vi "Sistema de ventilación-Ramirez.vi"() -> ()   [LabVIEW 2023]
uses:
  <vilib>/MakerHub/LINX/Public/Peripherals/Analog/Analog Read 1 Chan.vi
  <vilib>/MakerHub/LINX/Public/Peripherals/Digital/Digital Write 1 Chan.vi
  <vilib>/MakerHub/LINX/Public/Peripherals/Analog/Analog Read N Chans.vi
  <vilib>/MakerHub/LINX/Public/Peripherals/Digital/Digital Write N Chans.vi
  <vilib>/MakerHub/LINX/Private/Local IO/LinxAnalogRead.vi
  <vilib>/MakerHub/LINX/Public/Utilities/Check Channel.vi
  <vilib>/MakerHub/LINX/Private/Local IO/LinxDigitalWrite.vi
  <vilib>/MakerHub/LINX/Public/Utilities/Open Serial.vi
  <vilib>/MakerHub/LINX/Public/Sensors/Motion/Servo/Servo Open One Channel.vi
  <vilib>/MakerHub/LINX/Public/Peripherals/Analog/Analog Write 1 Chan.vi
  <vilib>/MakerHub/LINX/Private/Utilties/Generate Error.vi
  <vilib>/MakerHub/LINX/Public/Sensors/Motion/Servo/Servo Set Pulse Width One Channel.vi
  <vilib>/MakerHub/LINX/Public/Sensors/Motion/Servo/Servo Close One Channel.vi
  <vilib>/MakerHub/LINX/LMH-LINX.lvlib
  <vilib>/MakerHub/LINX/Public/Sensors/Motion/Servo/Servo.lvlib
panel:
  out "?":bool
  out "?":bool
  out "?":bool
  out "?":bool
  in  "?":bool
  out "Serevo Aire Angulo":string
  out "Serevo Temp Angulo":string
  in  "Serial Port":refnum<visa-resource-name>
  out "?":bool
  out "?":bool
  out "?":bool
  out "?":bool
  out "?":bool
  out "?":bool
  out "?":bool
  out "?":bool
  out "?":bool
  out "?":bool
  out "?":bool
  out "?":bool
  out "?":bool
  out "?":bool
  out "?":bool
  out "?":bool
  out "?":bool
  out "?":bool
  in  "?":bool
  out "Filtro de Calor":bool
  out "Filtro de Aire":bool
  out "Ppm del aire":dbl(knob) scale=0.0..1800.0
  out "Temperatura":dbl(slide) scale=0.0..60.0
  out "t [sec]":dbl
  out "Iteration No":i32
  in  "?":bool
  out "VI is running?":bool caption="ON/OFF"
  # "SISTEMA DE VENTILACIÓN DE DOBLE FLUJO"
  # "Temperatura"
  # "Entrada"
  # "Calidad del aire"
  # "Salida"
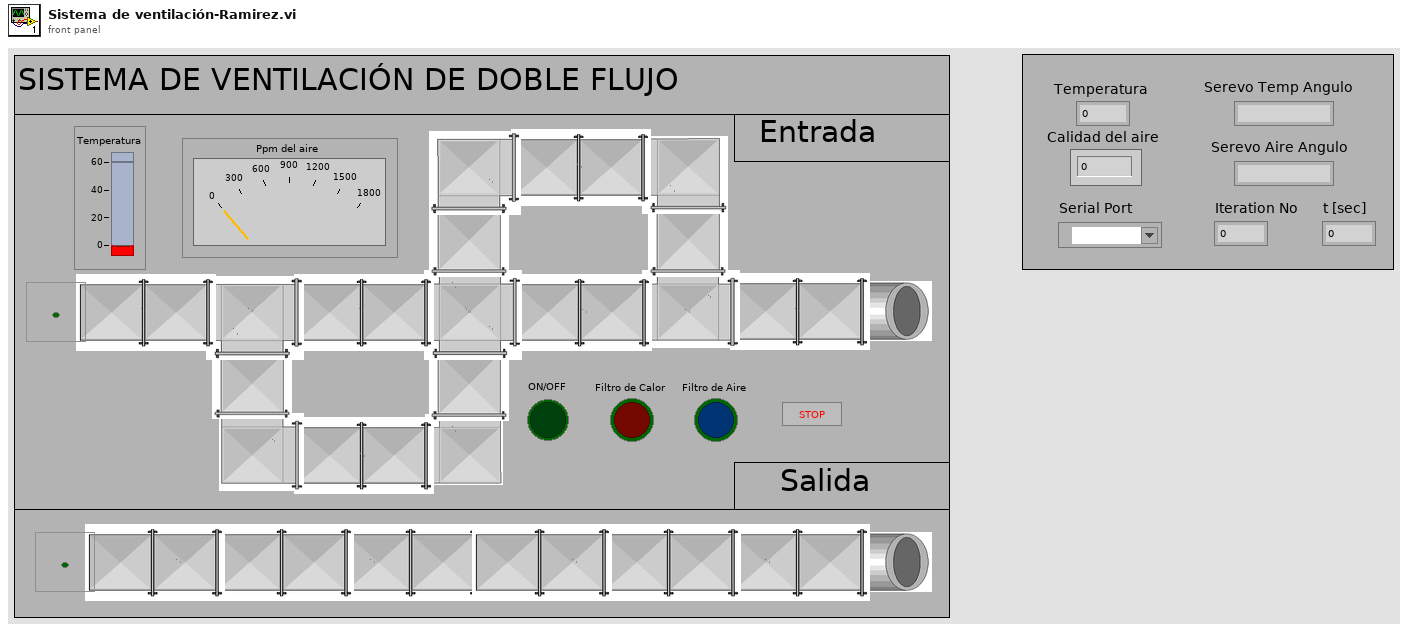
[diagram p1: front panel]
types:
  T1 = typedef "LMH-LINX.lvlib/LINX Ref.ctl" = cluster{"IO":T2, "Interface":T3, "LINX Device Config":T4}
  T2 = typedef "LMH-LINX.lvlib/Platform.ctl" = enum16{"Remote", "Local"}
  T3 = typedef "LMH-LINX.lvlib/Interface.ctl" = enum16{"Serial", "TCP"}
  T4 = typedef "LMH-LINX.lvlib/Device.lvlib/LINX Device Config.ctl" = cluster{"Interface":T3, "COM Port":refnum<visa-resource-name>, "TCP Configuration":T5, "Device Family":u8, "Device ID":u8, "Device Name":string, "TCP Ref":refnum<k5>, "Channels":T6}
  T5 = typedef "LMH-LINX.lvlib/Device.lvlib/TCP Config.ctl" = cluster{"IP Address":string, "Port":u16}
  T6 = typedef "LMH-LINX.lvlib/Channels.ctl" = cluster{"DI":u8[], "DO":u8[], "AI":u8[], "AO":u8[], "PWM":u8[], "QE":u8[], "UART":u8[], "I2C 2":u8[], "SPI":u8[], "CAN":u8[], "Servo":u8[], "AI Ref (V)":dbl, "AI Resolution (Bits)":u8, "AO Ref (V)":dbl, "AO Resolution (Bits)":u8}
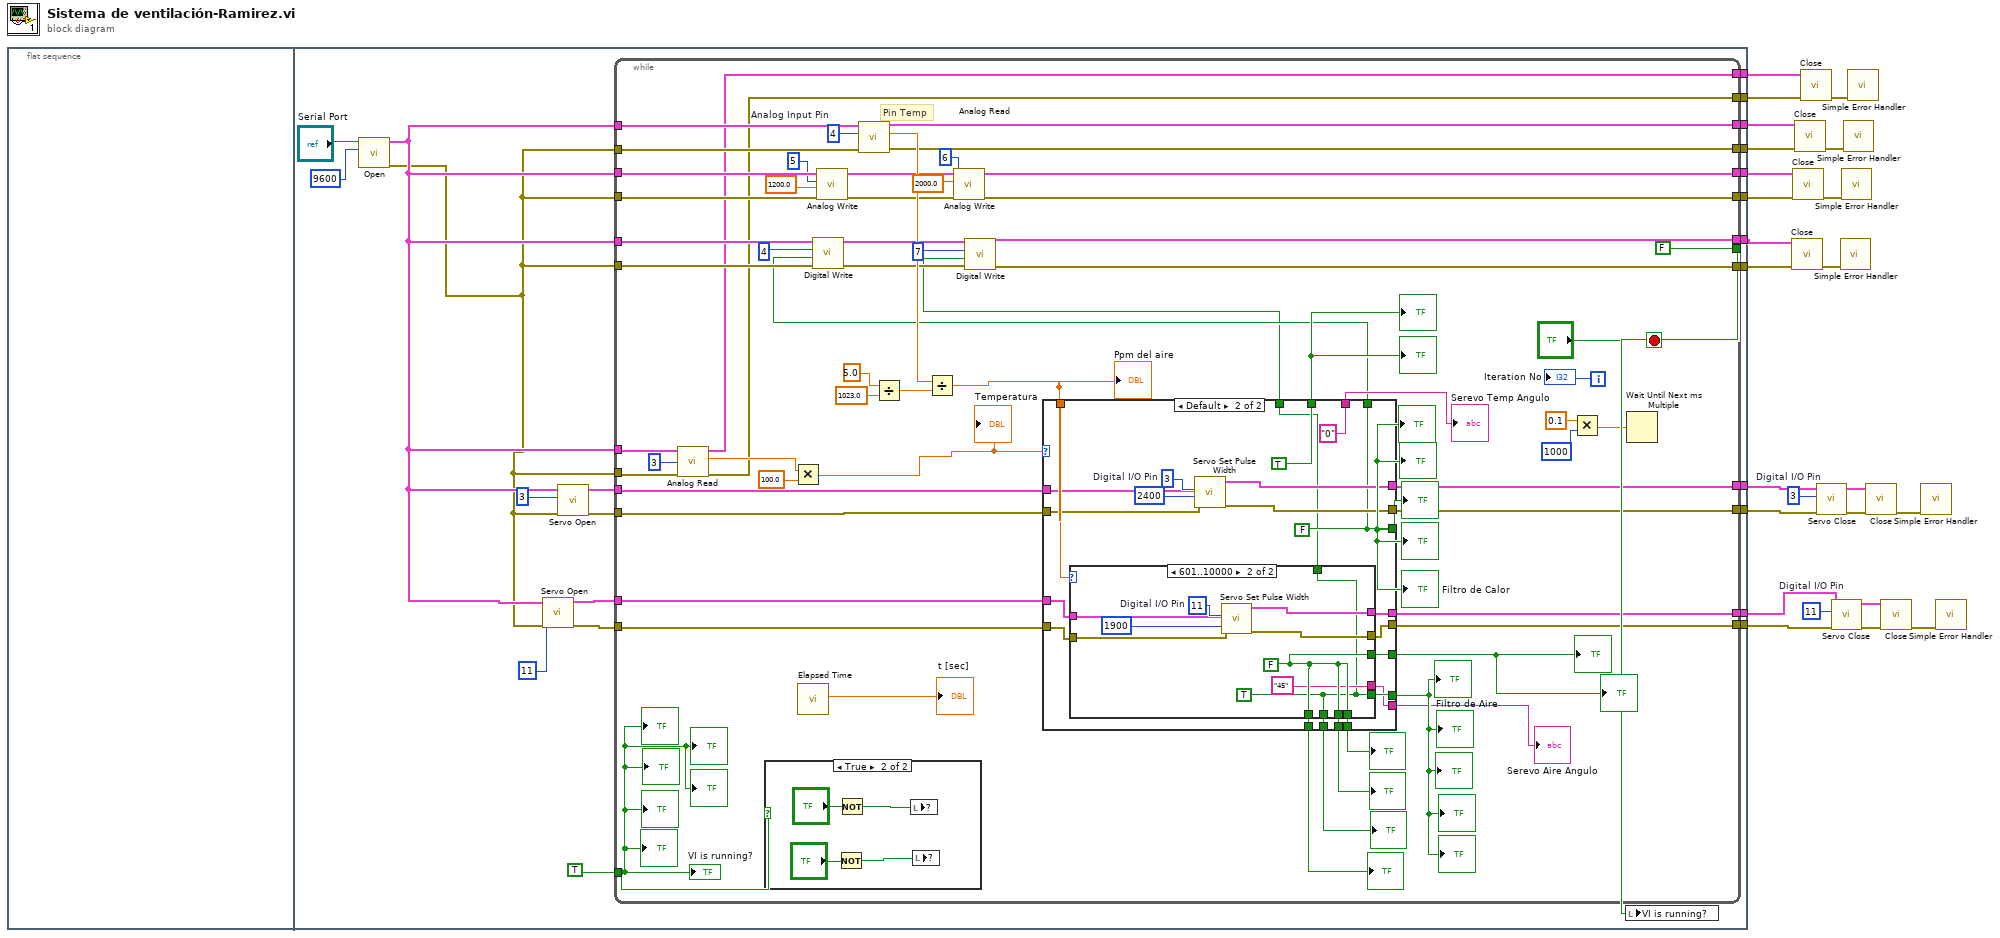
[diagram p0: block diagram]
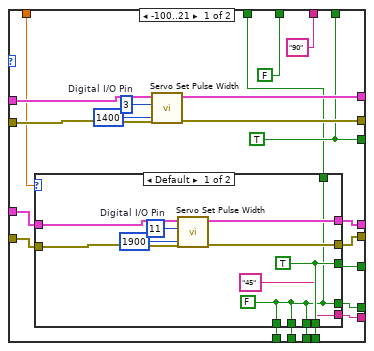
[diagram p2: hidden frame]
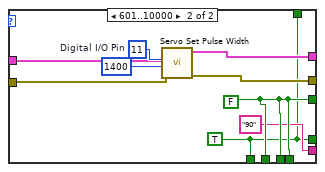
[diagram p3: hidden frame]
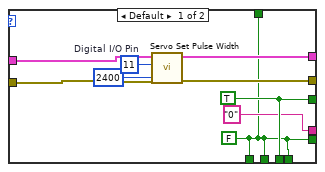
[diagram p4: hidden frame]
diagram:
  w7 = 11  # Digital I/O Pin
  w13 = 3  # Digital I/O Pin
  n1 = flat-sequence {
    tunnel: [w45] -> w24
    tunnel: [w43] -> w22
    tunnel: [w42] -> w20
    tunnel: [w41] -> w19
    tunnel: [w40] -> w17
    tunnel: [w39] -> w16
    tunnel: [w38] -> w1
    tunnel: [w37] -> w14
    tunnel: [w34] -> w9
    tunnel: [w33] -> w8
    tunnel: [w32] -> w3
    tunnel: [w31] -> w2
    frame #0 {
    }
    frame #1 {
      n2 = call-poly <vilib>:"Open.vi"("Baud Rate Override"=u32 9600, "Serial Port"="Serial Port") -> ("Error Out"=w27:errorcluster, "LINX Resource"=w29:T1)  [unwired: 7 in, 1 out]
      n3 = call-poly <vilib>:"Servo Open.vi"("Error In"=w27, "Servo Channel"=u8 11, "LINX Resource"=w29) -> ("Error Out"=w26:errorcluster, "LINX Resource"=w28:T1)  [unwired: 7 in]
      n4 = call-poly <vilib>:"Servo Open.vi"("Error In"=w27, "Servo Channel"=u8 3, "LINX Resource"=w29) -> ("Error Out"=w35:errorcluster, "LINX Resource"=w36:T1)  [unwired: 7 in]
      n5 = while {
        tunnel: [FALSE] -> w47
        tunnel: TRUE -> [w86]
        tunnel: w29 -> [w55]
        tunnel: [w57] -> w45
        tunnel: w27 -> [w54]
        tunnel: w29 -> [w105]
        tunnel: [w56] -> w43
        tunnel: w27 -> [w100]
        tunnel: [w98] -> w42
        tunnel: [w97] -> w41
        tunnel: w27 -> [w96]
        tunnel: w29 -> [w95]
        tunnel: [w88] -> w40
        tunnel: [w87] -> w39
        tunnel: w27 -> [w85]
        tunnel: w29 -> [w84]
        tunnel: [w79] -> w38
        tunnel: [w78] -> w37
        tunnel: w36 -> [w77]
        tunnel: w35 -> [w76]
        tunnel: [w75] -> w34
        tunnel: [w74] -> w33
        tunnel: w28 -> [w72]
        tunnel: w26 -> [w71]
        tunnel: [w70] -> w32
        tunnel: [w69] -> w31
        i -> [w107]
        stop <- "?" stop-if-true
        w99 = 4  # Analog Input Pin
        # "Pin Temp"
        n6 = call-poly <vilib>:"Analog Read.vi"("Error In"=w54, "Analog Channel"=u8 3, "LINX Resource"=w55) -> ("Error Out"=w56:errorcluster, "Voltage"=w58:dbl, "LINX Resource"=w57:T1)  [unwired: 5 in, 1 out]
        n7 = case shown="True" w86 {
          frame False {
          }
          frame True {
            n8 = Not(x="?") -> (.not. x?=w193:bool)
            n9 = Not(x="?") -> (.not. x?=w195:bool)
            n10 = local write item#8(w195) -> ()
            n11 = local write item#30(w193) -> ()
          }
        }
        n12 = Multiply(x=w58, y=100.0 ("x")) -> (x*y=w49:dbl)
        "Temperatura" <- w49
        n13 = call "Elapsed Time"() -> ("Elapsed Time (s)"=→"t [sec]":dbl)  [unwired: 12 in, 7 out]
        n14 = call-poly <vilib>:"Analog Write.vi"("Error In"=w96, "AO Value"=1200.0, "AO Channel"=5, "LINX Resource"=w95) -> ("Error Out"=w89:errorcluster, "LINX Resource"=w90:T1)  [unwired: 6 in]
        n15 = call-poly <vilib>:"Analog Read.vi"("Error In"=w100, "Analog Channel"=w99, "LINX Resource"=w105) -> ("Error Out"=w97:errorcluster, "Voltage"=w102:dbl, "LINX Resource"=w98:T1)  [unwired: 5 in, 1 out]
        n16 = Divide(x=5.0, y=1023.0) -> (x/y=w101:dbl)
        n17 = Divide(x=w102, y=w101) -> (x/y=w50:dbl)
        "Ppm del aire" <- w50
        n18 = call-poly <vilib>:"Analog Write.vi"("Error In"=w89, "AO Value"=2000.0, "AO Channel"=6, "LINX Resource"=w90) -> ("Error Out"=w88:errorcluster, "LINX Resource"=w87:T1)  [unwired: 6 in]
        n19 = case shown="Default" w49 {
          tunnel: w77 -> [w132 w172]
          tunnel: w76 -> [w131 w171]
          tunnel: [w130 w170] -> w75
          tunnel: [w129 w169] -> w74
          tunnel: [w114 w154] -> w73
          tunnel: [FALSE TRUE] -> w53
          tunnel: w72 -> [w124 w162]
          tunnel: w71 -> [w123 w161]
          tunnel: [w121 w163] -> w70
          tunnel: [w122 w164] -> w69
          tunnel: w50 -> [w125 w165]
          tunnel: [w127 w167] -> w68
          tunnel: [w126 w166] -> w67
          tunnel: [w120 w160] -> w66
          tunnel: [w117 w159] -> w65
          tunnel: [w118 w158] -> w64
          tunnel: [w119 w157] -> w63
          tunnel: ["90" ("Serevo Temp Angulo") "0" ("Serevo Temp Angulo")] -> w62
          tunnel: [w115 w155] -> w61
          tunnel: [w114 w154] -> w52
          tunnel: [w113 w153] -> w51
          frame -100..21 {
            w114 = TRUE
            w134 = 3  # Digital I/O Pin
            n20 = case shown="Default" w125 {
              tunnel: w124 -> [w141 w150]
              tunnel: w123 -> [w140 w149]
              tunnel: [w139 w148] -> w122
              tunnel: [w138 w147] -> w121
              tunnel: [w137 w146] -> w127
              tunnel: [w135 w144] -> w126
              tunnel: [w137 w146] -> w120
              tunnel: [w135 w144] -> w119
              tunnel: [w135 w146] -> w118
              tunnel: [w135 w146] -> w117
              tunnel: ["45" ("Serevo Aire Angulo") "90" ("Serevo Aire Angulo")] -> w115
              tunnel: [w135 w144] -> w113
              frame Default {
                w135 = FALSE
                w137 = TRUE
                w143 = 11  # Digital I/O Pin
                n21 = call-poly <vilib>:"Servo Set Pulse Width.vi"("Error In"=w140, "Pulse Width (uS)"=u16 1900, "Servo Channel"=w143, "LINX Resource"=w141) -> ("Error Out"=w138:errorcluster, "LINX Resource"=w139:T1)  [unwired: 6 in]
              }
              frame 601..10000 {
                w146 = FALSE
                w144 = TRUE
                w152 = 11  # Digital I/O Pin
                n22 = call-poly <vilib>:"Servo Set Pulse Width.vi"("Error In"=w149, "Pulse Width (uS)"=u16 1400, "Servo Channel"=w152, "LINX Resource"=w150) -> ("Error Out"=w147:errorcluster, "LINX Resource"=w148:T1)  [unwired: 6 in]
              }
            }
            n23 = call-poly <vilib>:"Servo Set Pulse Width.vi"("Error In"=w131, "Pulse Width (uS)"=u16 1400, "Servo Channel"=w134, "LINX Resource"=w132) -> ("Error Out"=w129:errorcluster, "LINX Resource"=w130:T1)  [unwired: 6 in]
          }
          frame Default {
            w154 = FALSE
            w174 = 3  # Digital I/O Pin
            n24 = case shown="601..10000" w165 {
              tunnel: w162 -> [w181 w191]
              tunnel: w161 -> [w180 w190]
              tunnel: [w179 w189] -> w164
              tunnel: [w178 w188] -> w163
              tunnel: [w177 w187] -> w167
              tunnel: [w175 w185] -> w166
              tunnel: [w175 w187] -> w160
              tunnel: [w177 w187] -> w159
              tunnel: [w175 w185] -> w158
              tunnel: [w175 w187] -> w157
              tunnel: ["0" ("Serevo Aire Angulo") "45" ("Serevo Aire Angulo")] -> w155
              tunnel: [w175 w185] -> w153
              frame Default {
                w175 = FALSE
                w177 = TRUE
                w183 = 11  # Digital I/O Pin
                n25 = call-poly <vilib>:"Servo Set Pulse Width.vi"("Error In"=w180, "Pulse Width (uS)"=u16 2400, "Servo Channel"=w183, "LINX Resource"=w181) -> ("Error Out"=w178:errorcluster, "LINX Resource"=w179:T1)  [unwired: 6 in]
              }
              frame 601..10000 {
                w187 = FALSE
                w185 = TRUE
                w192 = 11  # Digital I/O Pin
                n26 = call-poly <vilib>:"Servo Set Pulse Width.vi"("Error In"=w190, "Pulse Width (uS)"=u16 1900, "Servo Channel"=w192, "LINX Resource"=w191) -> ("Error Out"=w188:errorcluster, "LINX Resource"=w189:T1)  [unwired: 6 in]
              }
            }
            n27 = call-poly <vilib>:"Servo Set Pulse Width.vi"("Error In"=w171, "Pulse Width (uS)"=u16 2400, "Servo Channel"=w174, "LINX Resource"=w172) -> ("Error Out"=w169:errorcluster, "LINX Resource"=w170:T1)  [unwired: 6 in]
          }
        }
        "?" <- w64
        "?" <- w65
        "?" <- w63
        "?" <- w66
        "Serevo Temp Angulo" <- w62
        "Serevo Aire Angulo" <- w61
        "?" <- w73
        "?" <- w73
        "?" <- w73
        "?" <- w73
        "Filtro de Calor" <- w73
        "?" <- w53
        "?" <- w53
        "Filtro de Aire" <- w67
        "?" <- w67
        "?" <- w67
        "?" <- w67
        "?" <- w67
        "?" <- w68
        "?" <- w68
        n28 = call-poly <vilib>:"Digital Write.vi"("Error In"=w85, "Output Value"=w52, "DO Channel"=4, "LINX Resource"=w84) -> ("Error Out"=w80:errorcluster, "LINX Resource"=w81:T1)  [unwired: 6 in]
        n29 = call-poly <vilib>:"Digital Write.vi"("Error In"=w80, "Output Value"=w51, "DO Channel"=7, "LINX Resource"=w81) -> ("Error Out"=w78:errorcluster, "LINX Resource"=w79:T1)  [unwired: 6 in]
        n30 = Multiply(x=0.1, y=1000) -> (x*y=w110:dbl)
        n31 = Wait Until Next ms Multiple(millisecond multiple=w110) -> ()  [unwired: 1 out]
        "VI is running?" <- w86
        "Iteration No" <- w107
        "?" <- w86
        "?" <- w86
        "?" <- w86
        "?" <- w86
        "?" <- w86
        "?" <- w86
      }
      n32 = local write "VI is running?"(w47) -> ()
    }
  }
  n33 = call <vilib>:"Close.vi"("Error In"=w14, "LINX Resource"=w1) -> ("Error Out"=w15:errorcluster)  [unwired: 9 in]
  n34 = call <vilib>:"Close.vi"("Error In"=w17, "LINX Resource"=w16) -> ("Error Out"=w18:errorcluster)  [unwired: 9 in]
  n35 = call <vilib>:"Close.vi"("Error In"=w19, "LINX Resource"=w20) -> ("Error Out"=w21:errorcluster)  [unwired: 9 in]
  n36 = call <vilib>:"Close.vi"("Error In"=w22, "LINX Resource"=w24) -> ("Error Out"=w23:errorcluster)  [unwired: 9 in]
  n37 = call-poly <vilib>:"Servo Close.vi"("Error In"=w8, "Servo Channel"=w13, "LINX Resource"=w9) -> ("Error Out"=w11:errorcluster, "LINX Resource"=w12:T1)  [unwired: 7 in]
  n38 = call-poly <vilib>:"Servo Close.vi"("Error In"=w3, "Servo Channel"=w7, "LINX Resource"=w2) -> ("Error Out"=w5:errorcluster, "LINX Resource"=w6:T1)  [unwired: 7 in]
  n39 = call <vilib>:"Simple Error Handler.vi"("error in (no error)"=w15) -> ()  [unwired: 4 in, 5 out]
  n40 = call <vilib>:"Simple Error Handler.vi"("error in (no error)"=w18) -> ()  [unwired: 4 in, 5 out]
  n41 = call <vilib>:"Simple Error Handler.vi"("error in (no error)"=w21) -> ()  [unwired: 4 in, 5 out]
  n42 = call <vilib>:"Simple Error Handler.vi"("error in (no error)"=w23) -> ()  [unwired: 4 in, 5 out]
  n43 = call <vilib>:"Close.vi"("Error In"=w11, "LINX Resource"=w12) -> ("Error Out"=w10:errorcluster)  [unwired: 9 in]
  n44 = call <vilib>:"Close.vi"("Error In"=w5, "LINX Resource"=w6) -> ("Error Out"=w4:errorcluster)  [unwired: 9 in]
  n45 = call <vilib>:"Simple Error Handler.vi"("error in (no error)"=w10) -> ()  [unwired: 4 in, 5 out]
  n46 = call <vilib>:"Simple Error Handler.vi"("error in (no error)"=w4) -> ()  [unwired: 4 in, 5 out]
